vi "String 2 Signal.vi"(1 "String":string) -> (0 "Signal":dbl[](array[numeric]) format="%.2f")   [LabVIEW 2010]
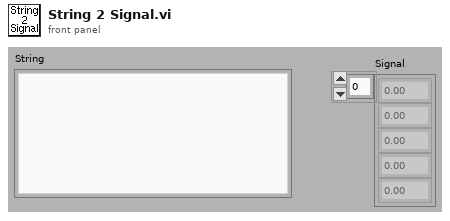
[diagram p1: front panel]
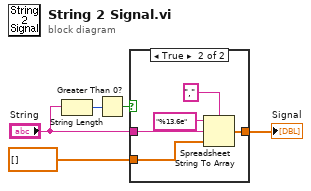
[diagram p0: block diagram]
diagram:
  n1 = String Length(string="String") -> (length=w3:i32)
  n2 = Greater Than 0?(x=w3) -> (x > 0?=w2:bool)
  n3 = case shown="True" w2 {
    tunnel: dbl[] [] ("Array Constant") -> [w6 w11]
    tunnel: "String" -> [_ w10]
    tunnel: [w6 w7] -> w4
    frame False {
    }
    frame True {
      n4 = Spreadsheet String To Array(delimiter (Tab)=",", format string="%13.6e", spreadsheet string=w10, array type (2D Dbl)=w11) -> (array=w7:dbl[])
    }
  }
  "Signal" <- w4
